vi "Show Nested Panel.vi"(8 "error in":errorcluster, 10 "Ident":string, 11 "Interactor in":refnum<class "Interactor.lvclass">) -> (0 "error out":errorcluster, 3 "Interactor out":refnum<class "Interactor.lvclass">)   [LabVIEW 2024, in "Interactor.lvlib" / "Interactor.lvclass"]
uses:
  Interactor.lvclass
  Interactor.lvclass/Interactor.ctl
  <vilib>/MGI/Panel Manager/Panel Actor/Panel Actor Messages/Show Panel Msg/Show Panel Msg.lvclass
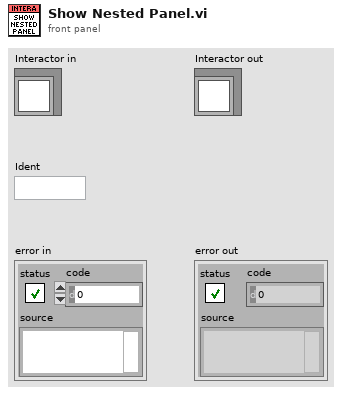
[diagram p1: front panel]
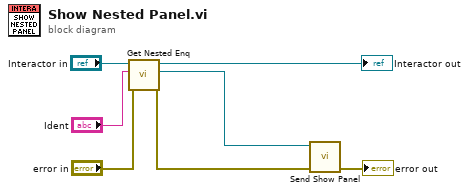
[diagram p0: block diagram]
diagram:
  n1 = call "Get Nested Enq.vi"("error in"="error in", "Ident"="Ident", "Interactor in"="Interactor in") -> ("error out"=w2:errorcluster, "Enq"=w1:refnum<class "Message Enqueuer.lvclass">, "Interactor out"=→"Interactor out":refnum<class "Interactor.lvclass">)  [unwired: 6 in]
  n2 = call <vilib>:"Send Show Panel.vi"("Error In"=w2, "Message Enqueuer in"=w1) -> ("Error Out"=→"error out":errorcluster)  [unwired: 8 in, 1 out]
